vi "constructCommand.vi"(8 "error in (no error)":errorcluster, 10 "commandValue":T1=enum."Start", 11 "SALCommunicator in":refnum<class "SALCommunicatorDL.lvclass">) -> (0 "error out":errorcluster, 3 "SALCommunicator out":refnum<class "SALCommunicatorDL.lvclass">)   [LabVIEW 2016, in "SALCommunicatorDL.lvclass"]
uses:
  SALCommunicatorDL.lvclass
  Typedefs/CommandValue.ctl
  SALCommunicatorDL.lvclass/SALCommunicatorDL.ctl
  CommandConstruction/CommandConstruction.lvclass
  SALCommand/StartSAL.lvclass
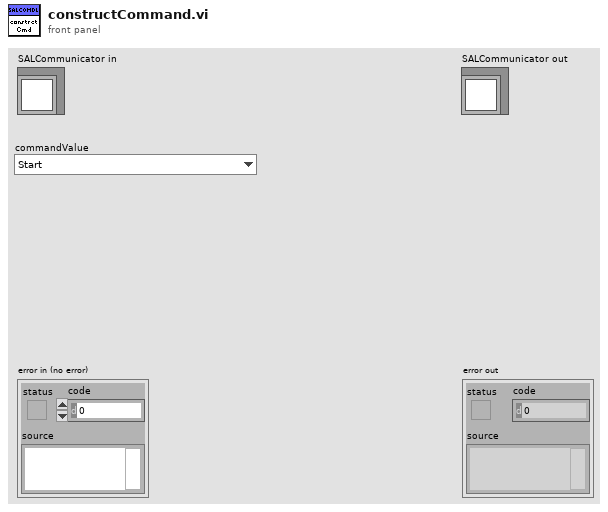
[diagram p1: front panel]
types:
  T1 = typedef "CommandValue.ctl" = enum16{"ClearError", "Disable", "Enable", "Exit", "GoToStandby", "OnHeartbeat", "OnIncomingMessagingError", "OnInterrupt", "Start"}
  T2 = typedef "SALLV_EXA.lvlib/command_start.ctl" = cluster{"configuration":string}
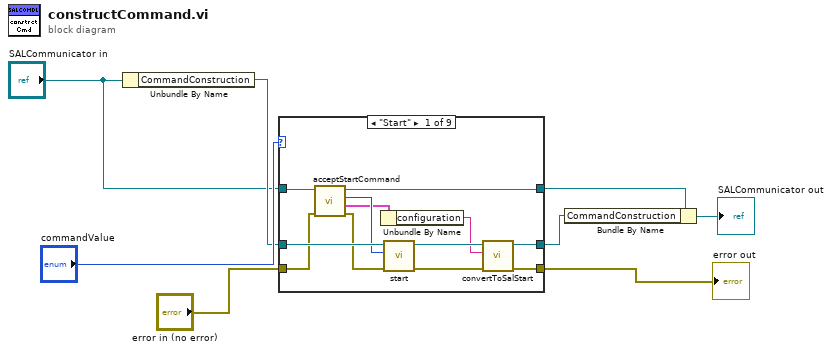
[diagram p0: block diagram]
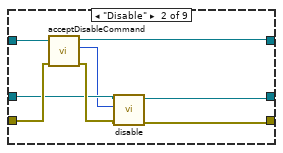
[diagram p2: hidden frame]
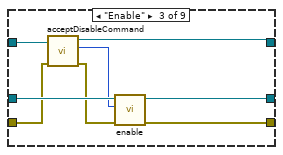
[diagram p3: hidden frame]
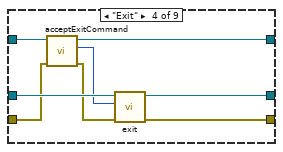
[diagram p4: hidden frame]
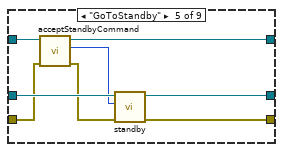
[diagram p5: hidden frame]
diagram:
  n1 = Unbundle By Name("SALCommunicator in") -> ("CommandConstruction"=w5:refnum<class "CommandConstruction.lvclass">)
  n2 = case shown="\"Start\"" "commandValue" {
    tunnel: "error in (no error)" -> [w18 w27 w32 w40 w49 w55 w58 w61 w64]
    tunnel: [w10 w24 w36 w44 w52 w55 w58 w61 w64] -> w6
    tunnel: w5 -> [w20 w22 w35 w43 w51 w54 w57 w60 w63]
    tunnel: [w11 w25 w34 w42 w50 w54 w57 w60 w63] -> w4
    tunnel: "SALCommunicator in" -> [w19 w28 w33 w41 w47 w53 w56 w59 w62]
    tunnel: [w15 w26 w29 w38 w46 w53 w56 w59 w62] -> w1
    frame "Start" {
      n3 = call "acceptStartCommand.vi"("error in (no error)"=w18, "SALCommunicator in"=w19) -> ("error out"=w17:errorcluster, "command_start_Ctl out"=w12:T2, "Command ID"=w16:i32, "SALCommunicator out"=w15:refnum<class "SALCommunicatorDL.lvclass">)  [unwired: 6 in]
      n4 = Unbundle By Name(w12) -> ("configuration"=w9:string)
      n5 = call "start.vi"("error in (no error)"=w17, "commandID"=w16, "CommandConstruction in"=w20) -> ("error out"=w14:errorcluster, "CommandConstruction out"=w13:refnum<class "CommandConstruction.lvclass">)  [unwired: 7 in]
      n6 = call "convertToSalStart.vi"("error in (no error)"=w14, "Configuration"=w9, "CommandConstruction in"=w13) -> ("error out"=w10:errorcluster, "CommandConstruction out"=w11:refnum<class "CommandConstruction.lvclass">)  [unwired: 7 in]
    }
    frame "Disable" {
      n7 = call "acceptDisableCommand.vi"("error in (no error)"=w27, "SALCommunicator in"=w28) -> ("error out"=w23:errorcluster, "Command ID"=w21:i32, "SALCommunicator out"=w26:refnum<class "SALCommunicatorDL.lvclass">)  [unwired: 7 in]
      n8 = call "disable.vi"("CommandConstruction in"=w22, "commandID"=w21, "error in (no error)"=w23) -> ("CommandConstruction out"=w25:refnum<class "CommandConstruction.lvclass">, "error out"=w24:errorcluster)  [unwired: 6 in]
    }
    frame "Enable" {
      n9 = call "acceptDisableCommand.vi"("error in (no error)"=w32, "SALCommunicator in"=w33) -> ("error out"=w31:errorcluster, "Command ID"=w30:i32, "SALCommunicator out"=w29:refnum<class "SALCommunicatorDL.lvclass">)  [unwired: 7 in]
      n10 = call "enable.vi"("error in (no error)"=w31, "Command ID"=w30, "CommandConstruction in"=w35) -> ("error out"=w36:errorcluster, "CommandConstruction out"=w34:refnum<class "CommandConstruction.lvclass">)  [unwired: 7 in]
    }
    frame "Exit" {
      n11 = call "acceptExitCommand.vi"("error in (no error)"=w40, "SALCommunicator in"=w41) -> ("error out"=w39:errorcluster, "Command ID"=w37:i32, "SALCommunicator out"=w38:refnum<class "SALCommunicatorDL.lvclass">)  [unwired: 7 in]
      n12 = call "exit.vi"("error in (no error)"=w39, "Command ID"=w37, "CommandConstruction in"=w43) -> ("error out"=w44:errorcluster, "CommandConstruction out"=w42:refnum<class "CommandConstruction.lvclass">)  [unwired: 7 in]
    }
    frame "GoToStandby" {
      n13 = call "acceptStandbyCommand.vi"("error in (no error)"=w49, "SALCommunicator in"=w47) -> ("error out"=w48:errorcluster, "Command ID"=w45:i32, "SALCommunicator out"=w46:refnum<class "SALCommunicatorDL.lvclass">)  [unwired: 7 in]
      n14 = call "standby.vi"("error in (no error)"=w48, "Command ID"=w45, "CommandConstruction in"=w51) -> ("error out"=w52:errorcluster, "CommandConstruction out"=w50:refnum<class "CommandConstruction.lvclass">)  [unwired: 7 in]
    }
    frame "OnHeartbeat" {
    }
    frame "OnIncomingMessagingError" {
    }
    frame "OnInterrupt" {
    }
    frame "ClearError" {
    }
  }
  "error out" <- w6
  n15 = Bundle By Name(cluster=w1, "CommandConstruction"=w4) -> (→"SALCommunicator out":refnum<class "SALCommunicatorDL.lvclass">)
